vi "duration.vi"(9 "seconds":dbl, 10 "minutes":dbl, 11 "hours":dbl) -> (3 "duration [s]":dbl)   [LabVIEW 2016]
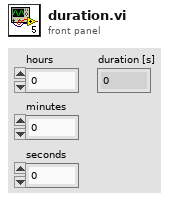
[diagram p1: front panel]
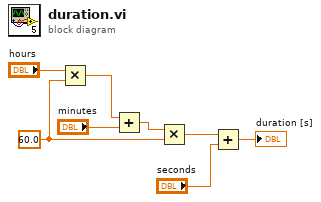
[diagram p0: block diagram]
diagram:
  w4 = 60.0
  n1 = Multiply(x="hours", y=w4) -> (x*y=w7:dbl)
  n2 = Add(x=w7, y="minutes") -> (x+y=w5:dbl)
  n3 = Multiply(x=w5, y=w4) -> (x*y=w3:dbl)
  n4 = Add(x=w3, y="seconds") -> (x+y=→"duration [s]":dbl)
